vi "Measurement UI.vi"() -> ()   [LabVIEW 2021, in "DAQmx Continuous Voltage Input.lvlib"]
uses:
  DAQmx Continuous Voltage Input.lvlib
  Typedef/Analog Pause.ctl
  Typedef/Analog Start.ctl
  Typedef/Waveform.ctl
panel:
  in  "Trigger Tab Enum":T1(ring)
  in  "Sample Clock Source str":string
  in  "Physical Channel str":string
  in  "TDMS File Path":path
  in  "Number of Samples":i32=100
  in  "Sample Rate":dbl=1000.0
  in  "Sample Clock Source":tag="OnboardClock"
  in  "Terminal Configuration":i32(ring)=-1 items=["default"=-1, "RSE"=10083, "NRSE"=10078, "Differential"=10106, "Pseudodifferential"=12529]
  in  "Max Voltage":dbl=5.0
  in  "Min Voltage":dbl=-5.0
  in  "Physical Channel":tag="Dev1/ai0"
  out "Actual Sample Rate":dbl=1000.0 format="%0.2f"
  in  "Logging Mode":i32(ring)=10231 items=["Off"=10231, "Log and Read"=15842]
  in  "Trigger Tab":T1(tab)
  in  "Digital Start Trigger Edge":i32(ring)=10280 caption="Edge" items=["Rising"=10280, "Falling"=10171]
  in  "Digital Start Trigger Source":tag="/Dev1/PFI0" caption="Source"
  in  "Digital Pause Trigger Pause When":i32(ring)=10192 caption="Pause When" items=["High"=10192, "Low"=10214]
  in  "Digital Pause Trigger Source":tag="/Dev1/PFI0" caption="Source"
  in  "Analog Start":T2={"Analog Start Trigger Source"="APFI0", "Analog Start Trigger Slope"=10280, "Analog Start Trigger Hysteresis"=0.0, "Analog Start Trigger Level"=0.0} {"Analog Start Trigger Level" format="%0.2f"; "Analog Start Trigger Hysteresis" format="%.2f"; "Analog Start Trigger Slope" items=["Rising"=10280, "Falling"=10171]}
  in  "Analog Pause":T3={"Analog Pause Trigger Source"="APFI0", "Analog Pause Trigger Pause When"=10093, "Analog Pause Trigger Level"=0.0} {"Analog Pause Trigger Level" format="%.2f"; "Analog Pause Trigger Pause When" items=["Above Level"=10093, "Below Level"=10107]}
  in  "When":timestamp
  in  "Select Time Manually":bool
  out "Waveform str":string
  in  "Digital Pause Source str":string
  in  "Digital Start Source str":string
  in  "Analog Pause str":string
  in  "Analog Start str":string
  in  "When str":string
  out "Waveform Graph":waveform(dbl)[](graph)
  # "Channel Settings"
  # "Timing Settings"
  # "Logging Settings"
  # "Trigger Settings"
  # "To enable triggers, select a tab above, and configure the settings.\n\nNot all hardware supports all trigger types. Refer to your device documentation for more information."
  # "This trigger type is not supported in continuous sample timing. \n\nRefer to your device documentation for more information on which triggers are supported."
  # "This trigger type is not supported in continuous sample timing. \n\nRefer to your device documentation for more information on which triggers are supported."
  # "If time is not manually set, task will begin after 10 seconds"
  # "Acquired Data"
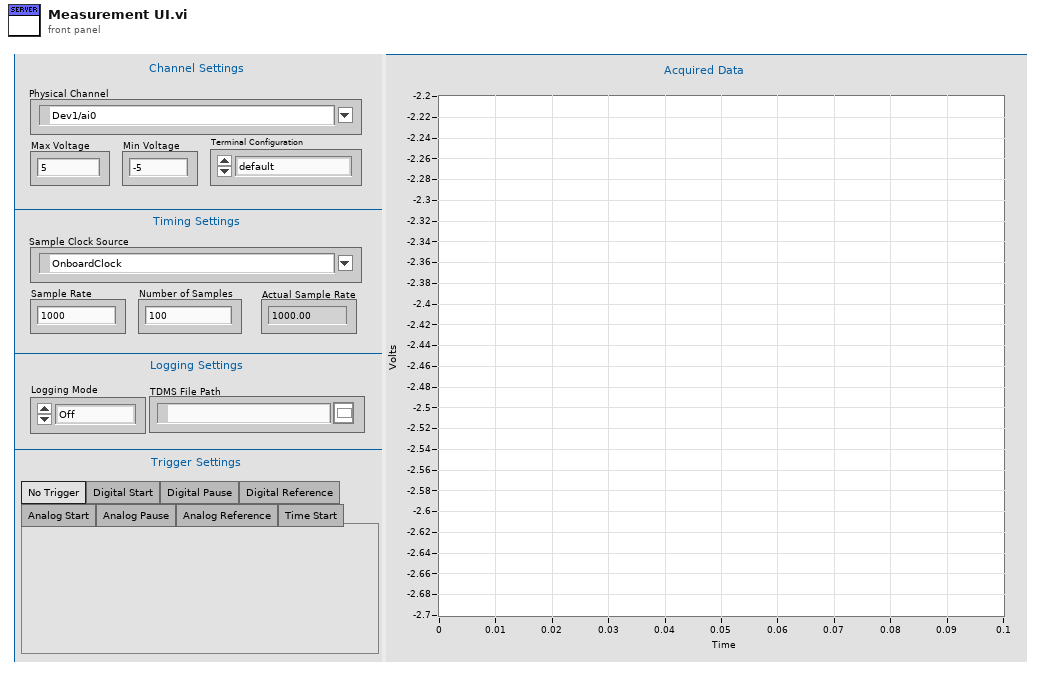
[diagram p1: front panel]
types:
  T1 = enum32{"No Trigger", "Digital Start", "Digital Pause", "Digital Reference", "Analog Start", "Analog Pause", "Analog Reference", "Time Start"}
  T2 = typedef "DAQmx Continuous Voltage Input.lvlib/Analog Start.ctl" = cluster{"Analog Start Trigger Source":string, "Analog Start Trigger Slope":i32, "Analog Start Trigger Hysteresis":dbl, "Analog Start Trigger Level":dbl}
  T3 = typedef "DAQmx Continuous Voltage Input.lvlib/Analog Pause.ctl" = cluster{"Analog Pause Trigger Source":string, "Analog Pause Trigger Pause When":i32, "Analog Pause Trigger Level":dbl}
  T4 = typedef "DAQmx Continuous Voltage Input.lvlib/Waveform.ctl" = cluster{"Y":dbl[], "dt":dbl}
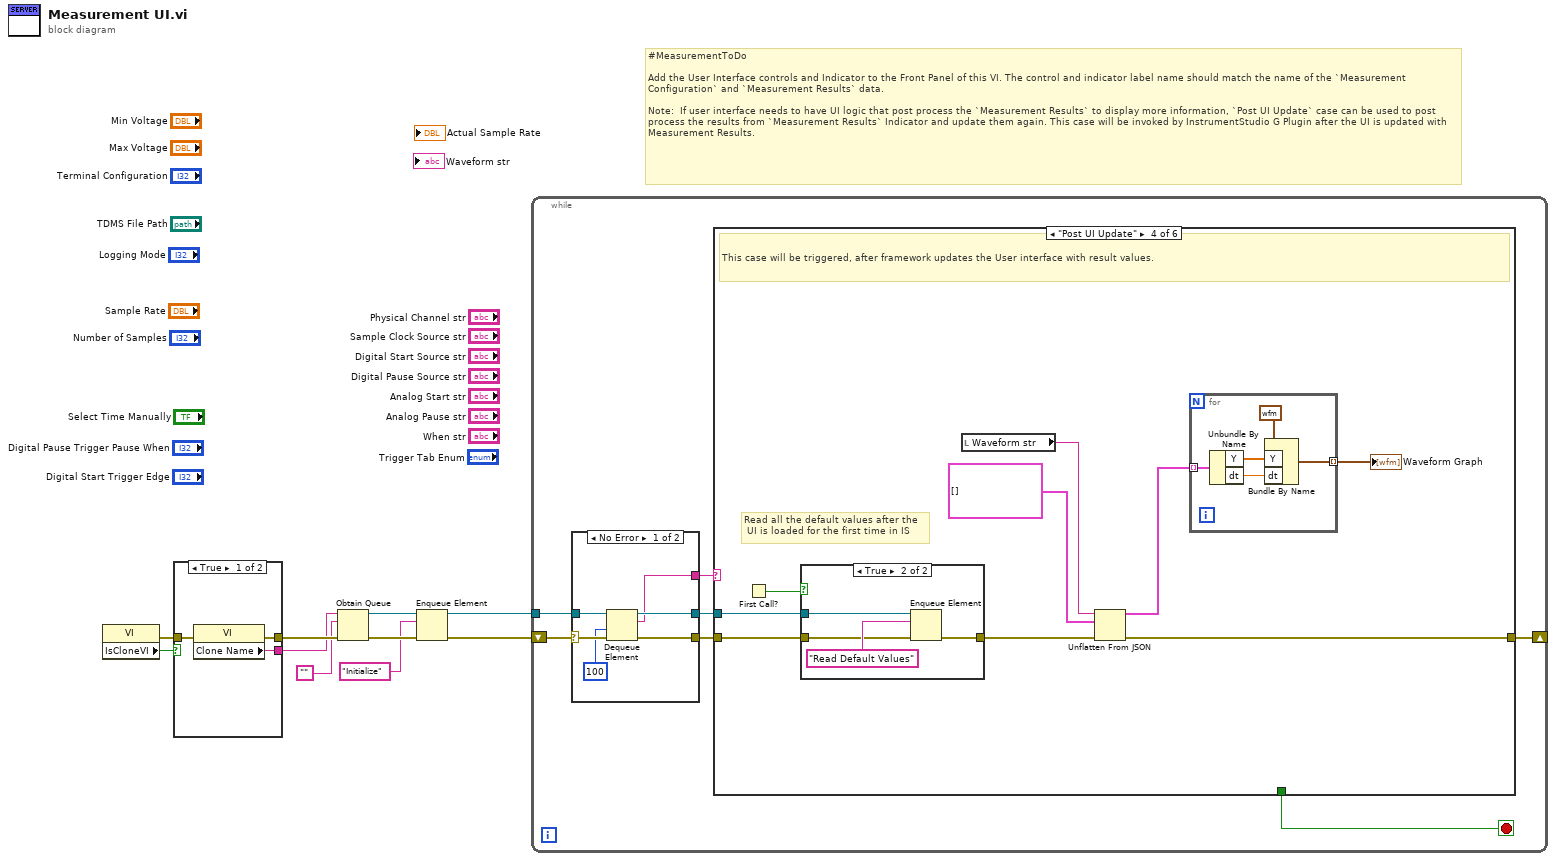
[diagram p0: block diagram]
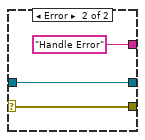
[diagram p2: hidden frame]
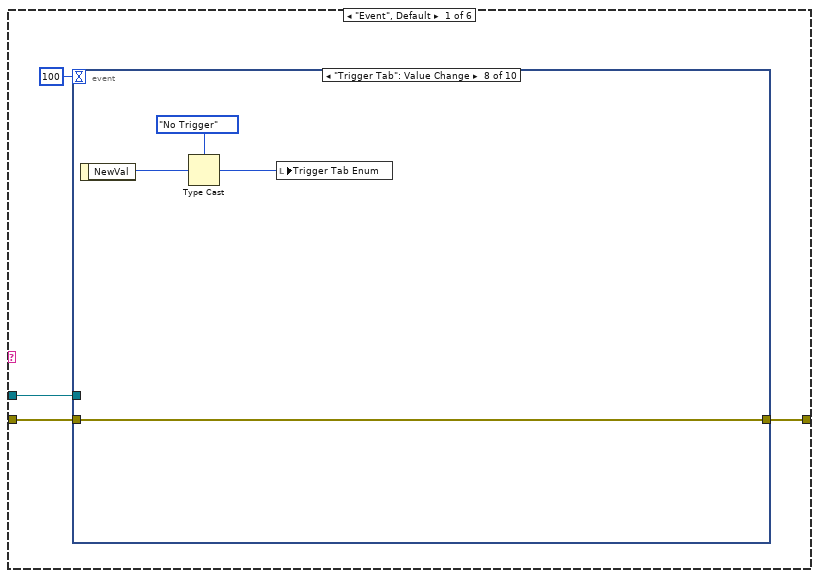
[diagram p3: hidden frame]
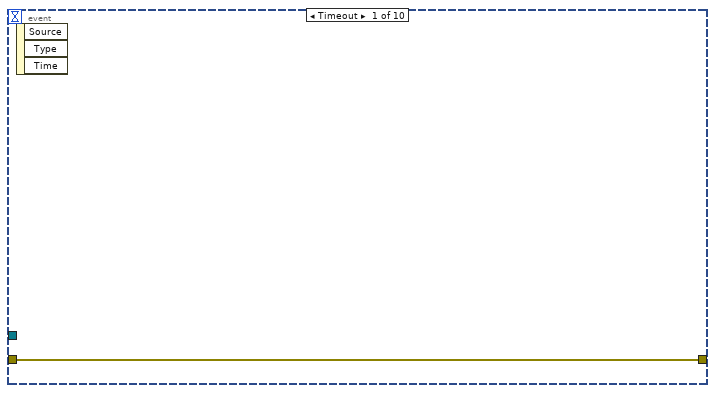
[diagram p4: hidden frame]
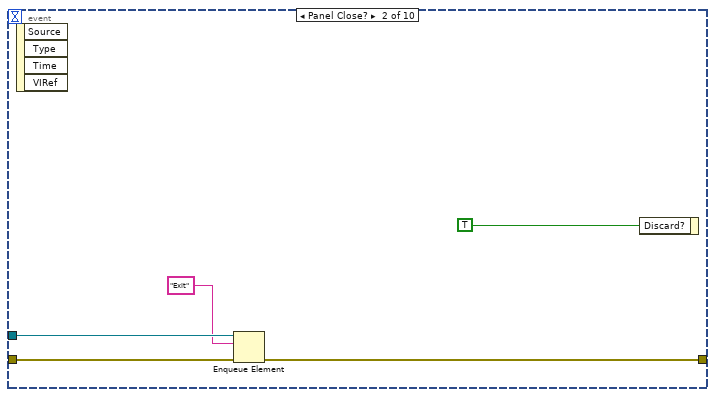
[diagram p5: hidden frame]
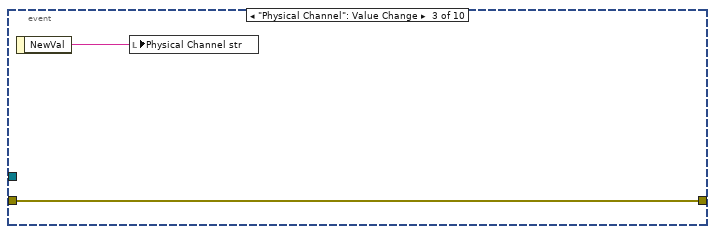
[diagram p6: hidden frame]
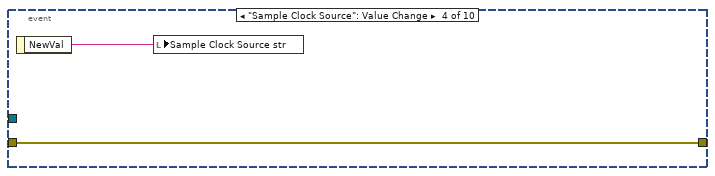
[diagram p7: hidden frame]
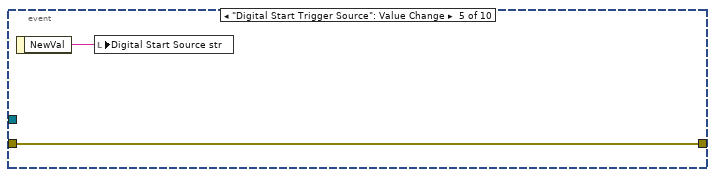
[diagram p8: hidden frame]
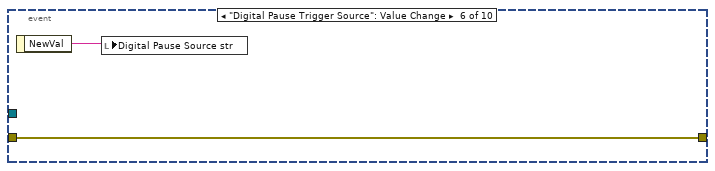
[diagram p9: hidden frame]
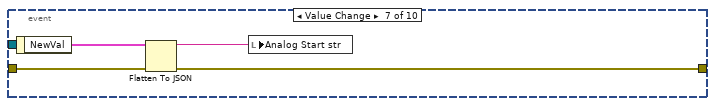
[diagram p10: hidden frame]
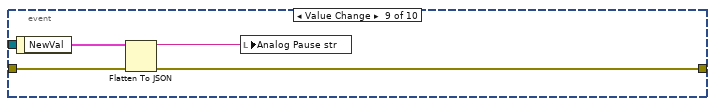
[diagram p11: hidden frame]
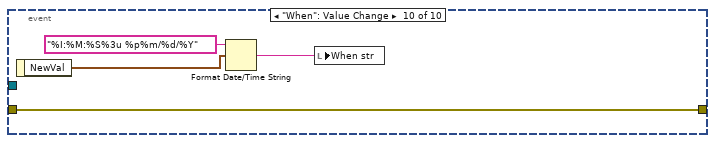
[diagram p12: hidden frame]
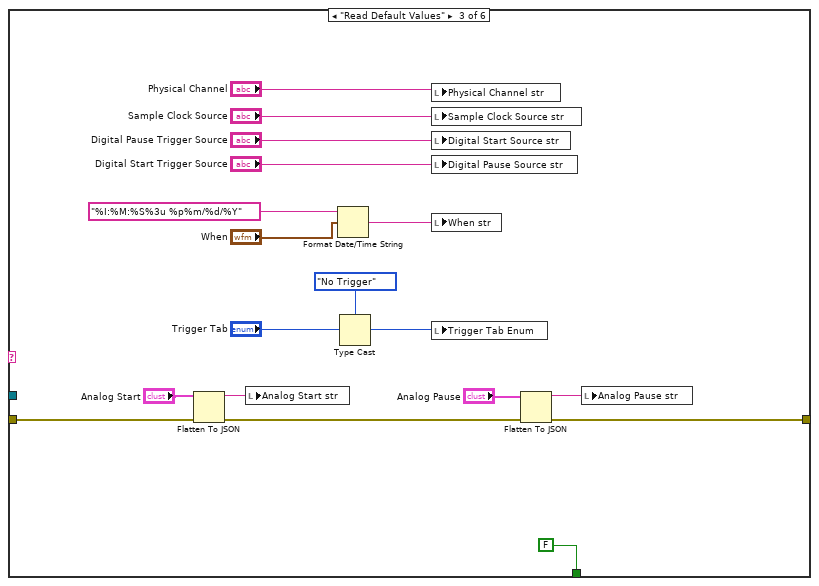
[diagram p14: hidden frame]
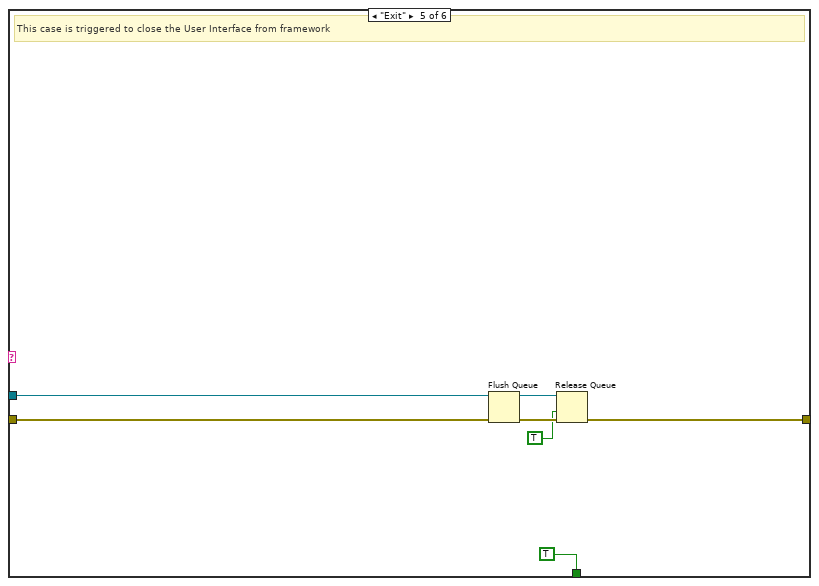
[diagram p16: hidden frame]
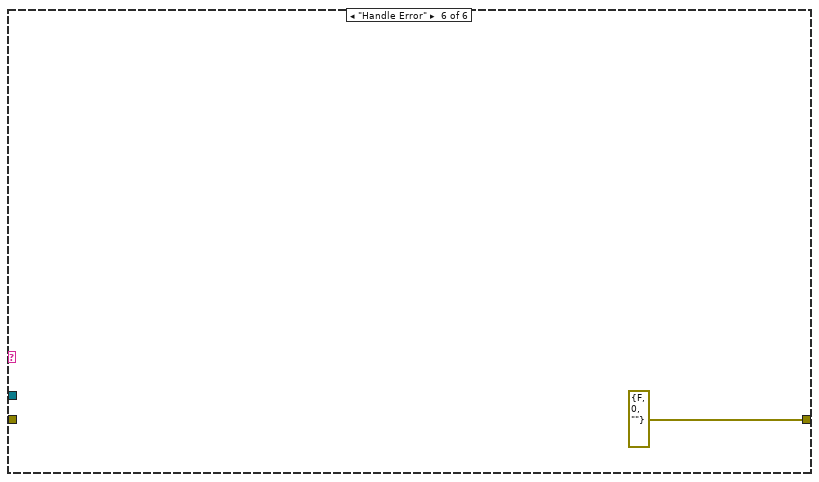
[diagram p17: hidden frame]
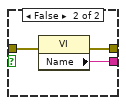
[diagram p18: hidden frame]
diagram:
  # "#MeasurementToDo  \n\nAdd the User Interface controls and Indicator to the Front Panel of this VI. The control and indicator label name should match the name of the `Measurement Configuration` and `Measurement Results` data.\n\nNote:  If user interface needs to have UI logic that post process the `Measurement Results` to display more information, `Post UI Update` case can be used to post process the results from `Measurement Results` Indicator and update them again. This case will be invoked by InstrumentStudio G Plugin after the UI is updated with Measurement Results."
  n1 = property class="VI"() -> (error out=w3:errorcluster, "IsCloneVI"=w4:bool)  [unwired: 2 in, 1 out]
  n2 = case shown="True" w4 {
    tunnel: [w13 w16] -> w10
    tunnel: [w12 w15] -> w9
    tunnel: w3 -> [w11 w14]
    frame True {
      n3 = property class="VI"(error in=w11) -> (error out=w13:errorcluster, "Clone Name"=w12:string)  [unwired: 1 in, 1 out]
    }
    frame False {
      n4 = property class="VI"(error in=w14) -> (error out=w16:errorcluster, "Name"=w15:string)  [unwired: 1 in, 1 out]
    }
  }
  n5 = Obtain Queue(name (unnamed)=w9, element data type="", error in (no error)=w10) -> (queue out=w7:refnum<queue>, error out=w8:errorcluster)  [unwired: 2 in, 1 out]
  n6 = Enqueue Element(queue=w7, element="Initialize", error in (no error)=w8) -> (queue out=w1:refnum<queue>, error out=w2:errorcluster)  [unwired: 1 in, 1 out]
  n7 = while {
    shift-right: [w20] -> _
    shift-left: w2 -> [w18]
    tunnel: w1 -> [w17]
    stop <- w19 stop-if-true
    n8 = case shown="No Error" w18 {
      selector: w18 -> [w29 w32]
      tunnel: [w28 w32] -> w23
      tunnel: w17 -> [w27 w31]
      tunnel: [w26 w31] -> w22
      tunnel: [w25 "Handle Error"] -> w21
      frame No Error {
        n9 = Dequeue Element(queue=w27, timeout in ms (-1)=100, error in (no error)=w29) -> (queue out=w26:refnum<queue>, element=w25:string, error out=w28:errorcluster)  [unwired: 1 out]
      }
      frame Error {
      }
    }
    n10 = case shown="\"Post UI Update\"" w21 {
      tunnel: w23 -> [w35 w67 w71 w87 w111 _]
      tunnel: w22 -> [w33 _ _ w89 w109 _]
      tunnel: [w36 w67 w69 w90 w106 errorcluster {"status"=FALSE, "code"=0, "source"=""} ("error out")] -> w20
      tunnel: [_ _ FALSE _ TRUE _] -> w19
      frame "Event", Default {
        n11 = event shown="[7] \"Trigger Tab\": Value Change" {
          selector: _ -> [_ _ _ _ _ _ _ _ _ _]
          dyn-events: _ -> [_ _ _ _ _ _ _ _ _ _]
          timeout: 100 -> [_ _ _ _ _ _ _ _ _ _]
          tunnel: [w37 w40 w44 w46 w48 w50 w52 w58 w61 w66] -> w36
          tunnel: w35 -> [w37 w41 w44 w46 w48 w50 w53 w58 w62 w66]
          tunnel: w33 -> [_ w39 _ _ _ _ _ _ _ _]
          event Timeout {
            n12 = event-data() -> ()  [unwired: 1 in, 3 out]
          }
          event Panel Close? {
            n13 = event-data() -> ()  [unwired: 1 in, 4 out]
            n14 = Enqueue Element(queue=w39, element="Exit", error in (no error)=w41) -> (error out=w40:errorcluster)  [unwired: 1 in, 2 out]
            n15 = event-data("Discard?"=TRUE) -> ()  [unwired: 1 in, 1 out]
          }
          event "Physical Channel": Value Change {
            n16 = event-data() -> ("NewVal"=w43:tag)  [unwired: 1 in]
            n17 = local write "Physical Channel str"(w43) -> ()
          }
          event "Sample Clock Source": Value Change {
            n18 = event-data() -> ("NewVal"=w45:tag)  [unwired: 1 in]
            n19 = local write "Sample Clock Source str"(w45) -> ()
          }
          event "Digital Start Trigger Source": Value Change {
            n20 = event-data() -> ("NewVal"=w47:tag)  [unwired: 1 in]
            n21 = local write "Digital Start Source str"(w47) -> ()
          }
          event "Digital Pause Trigger Source": Value Change {
            n22 = event-data() -> ("NewVal"=w49:tag)  [unwired: 1 in]
            n23 = local write "Digital Pause Source str"(w49) -> ()
          }
          event Value Change {
            n24 = event-data() -> ("NewVal"=w54:T2)  [unwired: 1 in]
            n25 = Flatten To JSON(anything=w54, error in (no error)=w53) -> (JSON string=w51:string, 11:w52:errorcluster)  [unwired: 1 in]
            n26 = local write "Analog Start str"(w51) -> ()
          }
          event "Trigger Tab": Value Change {
            n27 = event-data() -> ("NewVal"=w57:T1)  [unwired: 1 in]
            n28 = Type Cast(type=T1."No Trigger" ("Trigger Tab Enum"), x=w57) -> (*(type *) &x=w56:T1)
            n29 = local write "Trigger Tab Enum"(w56) -> ()
          }
          event Value Change {
            n30 = event-data() -> ("NewVal"=w60:T3)  [unwired: 1 in]
            n31 = Flatten To JSON(anything=w60, error in (no error)=w62) -> (JSON string=w59:string, 11:w61:errorcluster)  [unwired: 1 in]
            n32 = local write "Analog Pause str"(w59) -> ()
          }
          event "When": Value Change {
            n33 = event-data() -> ("NewVal"=w64:timestamp)  [unwired: 1 in]
            n34 = Format Date/Time String(time format string (%c)="%I:%M:%S%3u %p%m/%d/%Y", seconds (now)=w64) -> (date/time string=w63:string)  [unwired: 1 in]
            n35 = local write "When str"(w63) -> ()
          }
        }
      }
      frame "Initialize" {
      }
      frame "Read Default Values" {
        n36 = Flatten To JSON(anything="Analog Start", error in (no error)=w71) -> (JSON string=w79:string, 11:w70:errorcluster)  [unwired: 1 in]
        n37 = local write "Analog Start str"(w79) -> ()
        n38 = Format Date/Time String(time format string (%c)="%I:%M:%S%3u %p%m/%d/%Y", seconds (now)="When") -> (date/time string=w76:string)  [unwired: 1 in]
        n39 = Type Cast(type=T1."No Trigger" ("Trigger Tab Enum"), x="Trigger Tab") -> (*(type *) &x=w74:T1)
        n40 = local write "Physical Channel str"("Physical Channel") -> ()
        n41 = local write "Sample Clock Source str"("Sample Clock Source") -> ()
        n42 = local write "Digital Start Source str"("Digital Pause Trigger Source") -> ()
        n43 = local write "Digital Pause Source str"("Digital Start Trigger Source") -> ()
        n44 = local write "When str"(w76) -> ()
        n45 = local write "Trigger Tab Enum"(w74) -> ()
        n46 = Flatten To JSON(anything="Analog Pause", error in (no error)=w70) -> (JSON string=w72:string, 11:w69:errorcluster)  [unwired: 1 in]
        n47 = local write "Analog Pause str"(w72) -> ()
      }
      frame "Post UI Update" {
        # "Read all the default values after the\n UI is loaded for the first time in IS"
        # "This case will be triggered, after framework updates the User interface with result values."
        n48 = First Call?() -> (First Call?: T/F=w88:bool)
        n49 = case shown="True" w88 {
          tunnel: w89 -> [_ w98]
          tunnel: w87 -> [w95 w97]
          tunnel: [w95 w96] -> w86
          frame False {
          }
          frame True {
            n50 = Enqueue Element(queue=w98, element="Read Default Values", error in (no error)=w97) -> (error out=w96:errorcluster)  [unwired: 1 in, 2 out]
          }
        }
        n51 = local read "Waveform str"() -> (w93:string)
        n52 = Unflatten From JSON(JSON string=w93, type and defaults=T4[] [] ("Array"), error in (no error)=w86) -> (value=w91:T4[], error out=w90:errorcluster)  [unwired: 4 in]
        n53 = for {
          tunnel: [w104] -> w94 mode=indexing
          tunnel: w91 -> [w102] mode=indexing
          n54 = Unbundle By Name(w102) -> ("Y"=w101:dbl[], "dt"=w100:dbl)
          n55 = Bundle By Name(cluster=waveform(dbl) {"t0"=timestamp(0 s since 1904-01-01), "dt"=1.0, "Y"=[]}, "Y"=w101, "dt"=w100) -> (w104:waveform(dbl))
        }
        "Waveform Graph" <- w94
      }
      frame "Exit" {
        # "This case is triggered to close the User Interface from framework"
        n56 = Flush Queue(queue=w109, error in (no error)=w111) -> (queue out=w108:refnum<queue>, error out=w107:errorcluster)  [unwired: 1 out]
        n57 = Release Queue(queue=w108, force destroy? (F)=TRUE, error in (no error)=w107) -> (error out=w106:errorcluster)  [unwired: 2 out]
      }
      frame "Handle Error" {
      }
    }
  }
